vi "BC Async HP Data - RT-RT.vi"(8 "error in (no error)":errorcluster, 11 "Bus Controller in":refnum<class "Bus Controller.lvclass">) -> (0 "error out":errorcluster, 3 "Bus Controller out":refnum<class "Bus Controller.lvclass">)   [LabVIEW 2020, in "Unit Tests.lvlib" / "Bus Controller.lvclass"]
uses:
  Bus Controller.lvclass
  Frames & Messages/TypeDefs/Async Message Config.ctl
  Frames & Messages/TypeDefs/Command Config.ctl
  Frames & Messages/TypeDefs/Command Type.ctl
  Frames & Messages/TypeDefs/Command Terminal Address.ctl
  Frames & Messages/TypeDefs/Command SubAddress.ctl
  Frames & Messages/TypeDefs/Command Word Count.ctl
  Frames & Messages/TypeDefs/Message Control.ctl
  Frames & Messages/TypeDefs/Simplified Parameter Data Table.ctl
  Frames & Messages/TypeDefs/Scaling Information.ctl
  Frames & Messages/TypeDefs/Async RT-RT Message Config.ctl
  Bus Controller.lvclass/Bus Controller.ctl
  1553 Session/1553 Session.lvclass/1553 Session.ctl
  Bus Controller/Bus Controller.lvclass
  1553 Component/1553 Component.lvclass/1553 Component.ctl
  Frames & Messages/Async RT-RT Message/Async RT-RT Message.lvclass
  C:/Users/MattJ/Desktop/git/bci-1553-labview-api/src/Frames & Messages/Async Message/Async Message.lvclass
  <vilib>/addons/_JKI Toolkits/Caraya/classes/Assert/Assert True.vi
  1553 Component/1553 Component.lvclass
  1553 SubComponent/1553 SubComponent.lvclass
  Dependencies/FPGA Interface/FPGA Interface.lvclass
  BCI-1553 API.lvlib
  1553 Session/1553 Session.lvclass
  <vilib>/addons/_JKI Toolkits/Caraya/classes/Test/Test.lvclass
  <vilib>/addons/_JKI Toolkits/Caraya/classes/Assert/Assert.lvclass
panel:
  out "Data":u16[](array[numeric]) format="%04x"
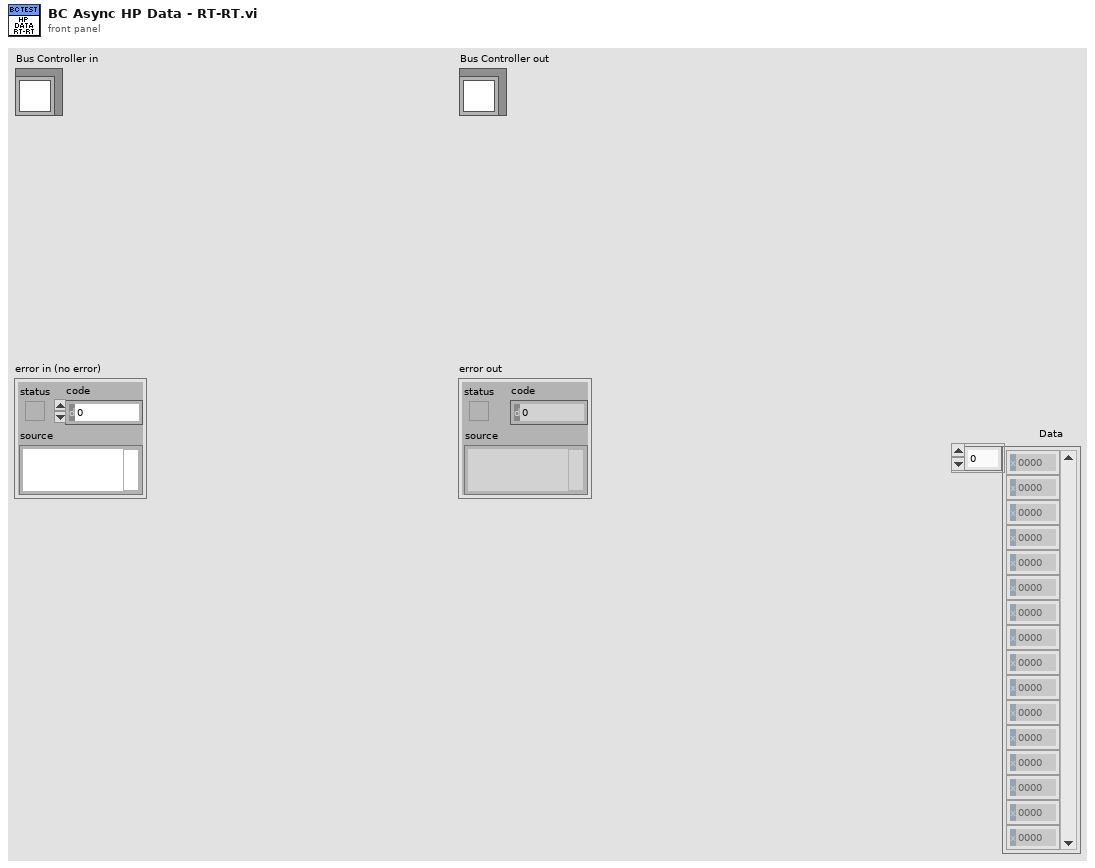
[diagram p1: front panel]
types:
  T1 = typedef "BCI-1553 API.lvlib/Command Word Count.ctl" = enum16{"1", "2", "3", "4", "5", "6", "7", "8", "9", "10", "11", "12", "13", "14", "15", "16", "17", "18", "19", "20", "21", "22", "23", "24", "25", "26", "27", "28", "29", "30", "31", "32"}
  T2 = typedef "BCI-1553 API.lvlib/Command SubAddress.ctl" = enum16{"Mode Code", "1", "2", "3", "4", "5", "6", "7", "8", "9", "10", "11", "12", "13", "14", "15", "16", "17", "18", "19", "20", "21", "22", "23", "24", "25", "26", "27", "28", "29", "30"}
  T3 = typedef "BCI-1553 API.lvlib/Command Terminal Address.ctl" = enum16{"0", "1", "2", "3", "4", "5", "6", "7", "8", "9", "10", "11", "12", "13", "14", "15", "16", "17", "18", "19", "20", "21", "22", "23", "24", "25", "26", "27", "28", "29", "30", "Broadcast"}
  T4 = typedef "BCI-1553 API.lvlib/Command Type.ctl" = enum16{"Transmit", "Receive"}
  T5 = typedef "BCI-1553 API.lvlib/Async RT-RT Message Config.ctl" = cluster{"Tx Command Config":T6}
  T6 = typedef "BCI-1553 API.lvlib/Command Config.ctl" = cluster{"Command Type":T4, "Terminal Address":T3, "SubAddress":T2, "Word Count\\Mode Code":T1, "Command Data":u16[]}
  T7 = typedef "BCI-1553 API.lvlib/Simplified Parameter Data Table.ctl" = cluster{"Parameter Name":string, "Base Word":u16, "Scaling Info":T8}
  T8 = typedef "BCI-1553 API.lvlib/Scaling Information.ctl" = cluster{"Bit Offset":i32, "Bit Count":i32, "LSB Resolution":dbl, "2's Complement":bool, "Big Endian":bool, "Sign Bit":bool}
  T9 = typedef "BCI-1553 API.lvlib/Async Message Config.ctl" = cluster{"Group":i32, "High Priority":bool, "Time to Next Msg (100 us)":u16, "Command Config":T6, "Message Control":T10}
  T10 = typedef "BCI-1553 API.lvlib/Message Control.ctl" = cluster{"MC17 Time Sync":bool, "Error Mask":bool, "Service Request Mask":bool, "Busy Mask":bool, "SubSystem Flag Mask":bool, "Terminal Flag Mask":bool, "Reserved Mask":bool, "Retry":bool, "Bus A / !Bus B":bool, "Self-Test Loopback":bool, "Broadcast Mask":bool, "EoM Interrupt":bool, "Mode Code Format":bool, "Broadcast Format":bool, "RT-RT Format":bool}
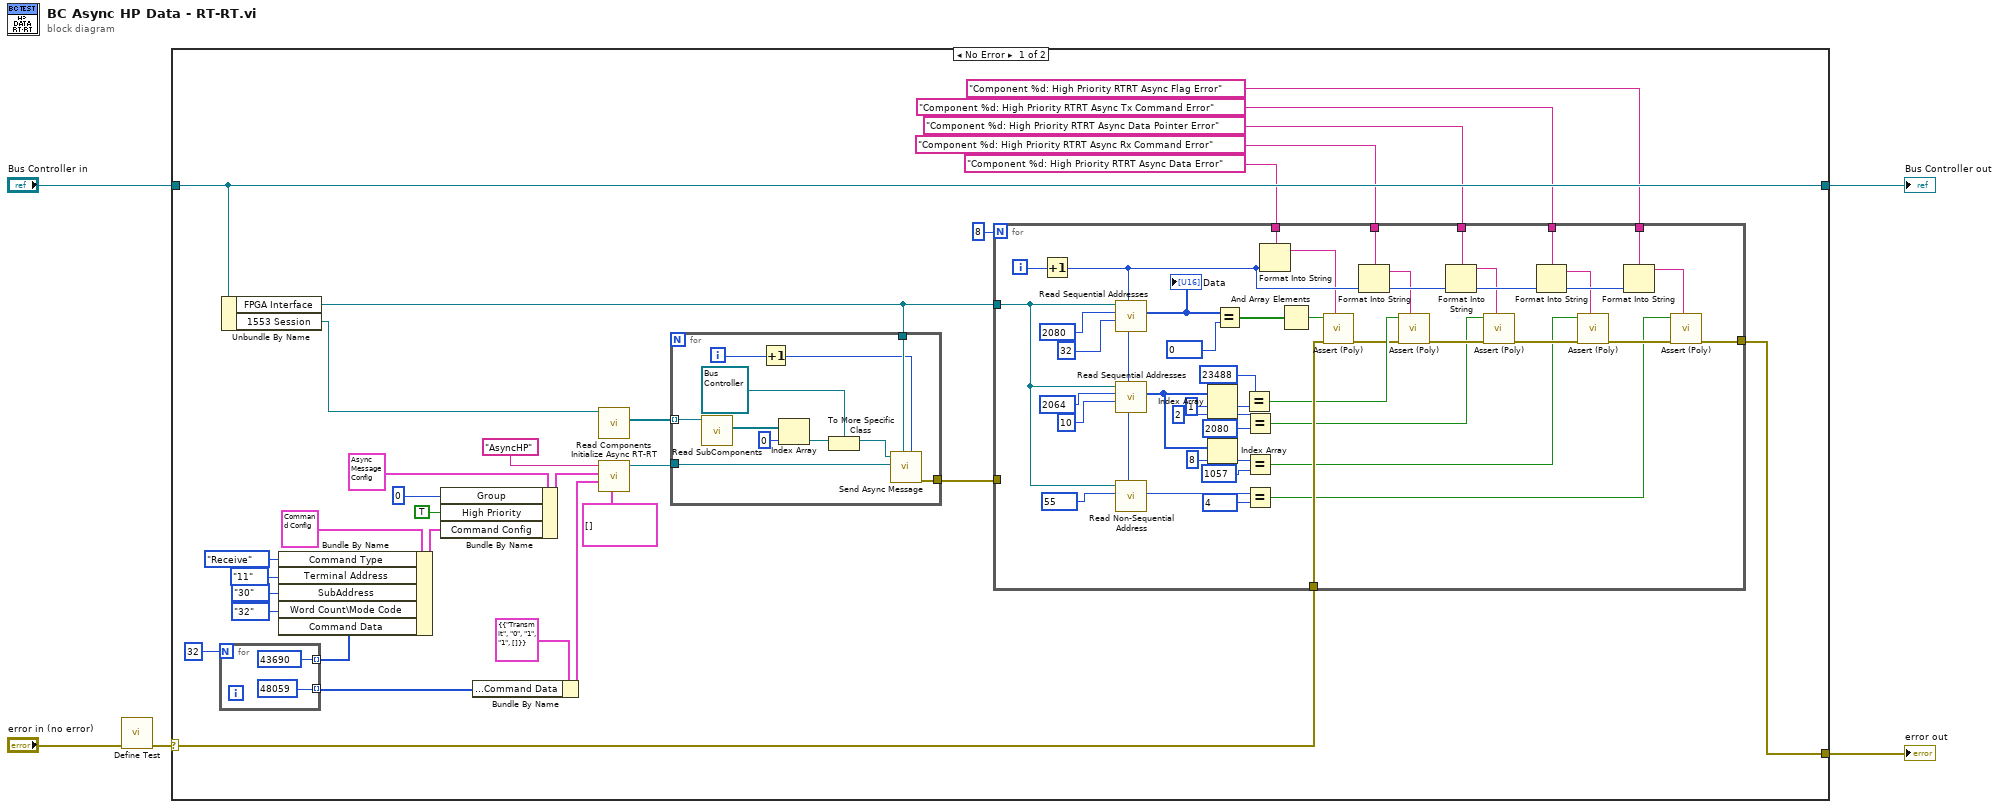
[diagram p0: block diagram]
diagram:
  n1 = call <vilib>:"Define Test.vi"("error in (no error)"="error in (no error)") -> ("error out"=w2:errorcluster)  [unwired: 9 in, 1 out]
  n2 = case shown="No Error" w2 {
    selector: w2 -> [w19 w95]
    tunnel: [w18 w95] -> w5
    tunnel: [w36 w94] -> w3
    tunnel: "Bus Controller in" -> [w36 w94]
    frame No Error {
      n3 = for {
        N: 32 -> [_]
        tunnel: [u16 43690] -> w29 mode=indexing
        tunnel: [u16 48059] -> w26 mode=indexing
      }
      n4 = Unbundle By Name(w36) -> ("FPGA Interface"=w21:refnum<class "FPGA Interface.lvclass">, "1553 Session"=w23:refnum<class "1553 Session.lvclass">)
      n5 = Bundle By Name(cluster=T6 {"Command Type"=enum."Transmit", "Terminal Address"=enum."0", "SubAddress"=enum."Mode Code", "Word Count\\Mode Code"=enum."1", "Command Data"=[]} ("Command Config"), "Command Type"=Command_Type."Receive", "Terminal Address"=Command_Terminal_Address."11", "SubAddress"=Command_SubAddress."30", "Word Count\\Mode Code"=Command_Word_Count."32" ("Word Count\\Mode Code"), "Command Data"=w29) -> (w32:T6)
      n6 = Bundle By Name(cluster=T9 {"Group"=0, "High Priority"=FALSE, "Time to Next Msg (100 us)"=0, "Command Config"={"Command Type"=enum."Transmit", "Terminal Address"=enum."0", "SubAddress"=enum."Mode Code", "Word Count\\Mode Code"=enum."1", "Command Data"=[]}, "Message Control"={"MC17 Time Sync"=FALSE, "Error Mask"=FALSE, "Service Request Mask"=FALSE, "Busy Mask"=FALSE, "SubSystem Flag Mask"=FALSE, "Terminal Flag Mask"=FALSE, "Reserved Mask"=FALSE, "Retry"=FALSE, "Bus A / !Bus B"=FALSE, "Self-Test Loopback"=FALSE, "Broadcast Mask"=FALSE, "EoM Interrupt"=FALSE, "Mode Code Format"=FALSE, "Broadcast Format"=FALSE, "RT-RT Format"=FALSE}} ("Async Message Config"), "Group"=0, "High Priority"=TRUE, "Command Config"=w32) -> (w27:T9)
      n7 = Bundle By Name(cluster=T5 {"Tx Command Config"={"Command Type"=enum."Transmit", "Terminal Address"=enum."0", "SubAddress"=enum."1", "Word Count\\Mode Code"=enum."1", "Command Data"=[]}} ("Transmit Message Config"), "Tx Command Config.Command Data"=w26) -> (w10:T5)
      n8 = call "Read Components.vi"("1553 Board in"=w23) -> ("Components"=w22:refnum<class "1553 Component.lvclass">[])  [unwired: 8 in, 2 out]
      n9 = call "Initialize Async RT-RT.vi"("Parameters"=T7[] [], "Transmit Message Config"=w10, "Receive Message Config"=w27, "ID"="AsyncHP") -> ("Async RT-RT Message out"=w24:refnum<class "Async RT-RT Message.lvclass">)  [unwired: 6 in, 1 out]
      n10 = for {
        tunnel: w22 -> [w91] mode=indexing
        tunnel: w24 -> [w85]
        tunnel: w21 -> [w84]
        tunnel: [w81] -> w20
        i -> [w83]
        n11 = call "Read SubComponents.vi"("1553 Component in"=w91) -> ("SubComponents"=w90:refnum<class "1553 SubComponent.lvclass">[])  [unwired: 8 in, 2 out]
        n12 = Increment(x=w83) -> (x+1=w82:i32)
        n13 = Index Array(array=w90, index=0) -> (element=w88:refnum<class "1553 SubComponent.lvclass">)
        n14 = To More Specific Class(target class=refnum<class "Bus Controller.lvclass"> refnum ("SLSC 1553 API.lvlib:Bus Controller.lvclass"), reference=w88) -> (specific class reference=w86:refnum<class "Bus Controller.lvclass">)  [unwired: 1 in, 1 out]
        n15 = call-dynamic "Send Async Message.vi"("Component ID"=w82, "FPGA Interface"=w84, "Async Message"=w85, "Bus Controller in"=w86) -> ("error out"=w81:errorcluster)  [unwired: 6 in, 1 out]
      }
      n16 = for {
        N: 8 -> [_]
        tunnel: w21 -> [w66]
        tunnel: w19 -> [w50]
        tunnel: [w37] -> w18
        tunnel: "Component %d: High Priority RTRT Async Data Error" ("custom report message (\"\")") -> [w79]
        tunnel: "Component %d: High Priority RTRT Async Rx Command Error" ("custom report message (\"\")") -> [w64]
        tunnel: "Component %d: High Priority RTRT Async Data Pointer Error" ("custom report message (\"\")") -> [w63]
        tunnel: "Component %d: High Priority RTRT Async Flag Error" ("custom report message (\"\")") -> [w62]
        tunnel: "Component %d: High Priority RTRT Async Tx Command Error" ("custom report message (\"\")") -> [w53]
        tunnel: w20 -> [_]
        i -> [w80]
        n17 = Increment(x=w80) -> (x+1=w54:i32)
        n18 = call-dynamic "Read Sequential Addresses.vi"("Target IC (1-8)"=w54, "Addresses to Read"=u16 32, "Starting Address"=u16 2080, "FPGA Interface in"=w66) -> ("Data"=w74:u16[])  [unwired: 6 in, 1 out]
        "Data" <- w74
        n19 = call-dynamic "Read Sequential Addresses.vi"("Target IC (1-8)"=w54, "Addresses to Read"=u16 10, "Starting Address"=u16 2064, "FPGA Interface in"=w66) -> ("Data"=w58:u16[])  [unwired: 6 in, 1 out]
        n20 = call-dynamic "Read Non-Sequential Address.vi"("Target IC (1-8)"=w54, "Address"=u16 55, "FPGA Interface in"=w66) -> ("Data"=w59:u16)  [unwired: 7 in, 1 out]
        n21 = Index Array(array=w58, index #1=1 ("index"), index #2=2 ("index")) -> (element #1=w68:u16, element #2=w60:u16)
        n22 = Index Array(array=w58, index=8) -> (element=w56:u16)
        n23 = Equal?(x=w74, y=u16 0) -> (x = y?=w72:bool[])
        n24 = Equal?(x=u16 23488, y=w68) -> (x = y?=w49:bool)
        n25 = Equal?(x=w60, y=u16 2080) -> (x = y?=w44:bool)
        n26 = Equal?(x=w56, y=u16 1057) -> (x = y?=w41:bool)
        n27 = Equal?(x=w59, y=u16 4) -> (x = y?=w39:bool)
        n28 = Format Into String(format string=w79, w54) -> (resulting string=w51:string)  [unwired: 2 in, 1 out]
        n29 = And Array Elements(Boolean array=w72) -> (logical AND=w52:bool)
        n30 = call-poly <vilib>:"Assert (Poly).vi"("Label"=w51, "error in (no error)"=w50, "True?"=w52) -> ("error out"=w48:errorcluster)  [unwired: 7 in, 1 out]
        n31 = Format Into String(format string=w64, w54) -> (resulting string=w47:string)  [unwired: 2 in, 1 out]
        n32 = call-poly <vilib>:"Assert (Poly).vi"("Label"=w47, "error in (no error)"=w48, "True?"=w49) -> ("error out"=w46:errorcluster)  [unwired: 7 in, 1 out]
        n33 = Format Into String(format string=w63, w54) -> (resulting string=w45:string)  [unwired: 2 in, 1 out]
        n34 = call-poly <vilib>:"Assert (Poly).vi"("Label"=w45, "error in (no error)"=w46, "True?"=w44) -> ("error out"=w43:errorcluster)  [unwired: 7 in, 1 out]
        n35 = Format Into String(format string=w53, w54) -> (resulting string=w42:string)  [unwired: 2 in, 1 out]
        n36 = call-poly <vilib>:"Assert (Poly).vi"("Label"=w42, "error in (no error)"=w43, "True?"=w41) -> ("error out"=w40:errorcluster)  [unwired: 7 in, 1 out]
        n37 = Format Into String(format string=w62, w54) -> (resulting string=w38:string)  [unwired: 2 in, 1 out]
        n38 = call-poly <vilib>:"Assert (Poly).vi"("Label"=w38, "error in (no error)"=w40, "True?"=w39) -> ("error out"=w37:errorcluster)  [unwired: 7 in, 1 out]
      }
    }
    frame Error {
    }
  }
  "error out" <- w5
  "Bus Controller out" <- w3
